vi "Turret Controller.vi"(8 "error in":errorcluster) -> ()   [LabVIEW 2019]
doc: "This VI executes continuously carrying out the current operation and responding to updates or new operations. It will often contain the timing or control code that is difficult to place directly in TeleOp. This VI generally opens all sensors and motors and isolates the rest of the robot code from knowing how the operations are carried out."
uses:
  <vilib>/Rock Robotics/WPI/Framework/Completion Status.ctl
  Turret Setpoints.ctl
  Turret Operations.ctl
  <vilib>/Rock Robotics/SystemInterfaces/DIO/FPGA_DIOChannel.ctl
  <vilib>/Rock Robotics/WPI/ThirdParty/REV Robotics/SPARK MAX/Typedef/Spark MAX Control Type.ctl
  Turret Published Globals.vi
  Framework/Robot Global Data.vi
  <vilib>/addons/control/pid/pid.llb/PID (DBL).vi
  <vilib>/addons/control/pid/NI_PID_pid.lvlib
  <vilib>/Rock Robotics/Network Tables/NT Write Boolean.vi
panel:
  out "Sensor Position 2":dbl
  out "Hood Position":T1(graph)
  out "Sensor Position":dbl
  out "Turret Position":T1(graph)
  out "Turret Position":cluster{"output":dbl, "Horizontal Offset":dbl}(graph)
  in  "DIO Channels":cluster{"Turret Encoder":T2, "Hood Encoder":T2}={"Turret Encoder"=enum."DIO 0", "Hood Encoder"=enum."DIO 1"}
  in  "Motor CAN IDs":T3={"Shooter Left"=12, "Shooter Right"=13, "Turret"=10, "Hood"=14}
  out "Setpoints":T4(graph)
  in  "Interactive Values":T5
  out "Current\nCmd":string
  in  "Buttons":cluster{"Execute Cmd":bool, "Abort Cmd":bool}
  out "Command Timing":cluster{"Start Time (ms)":u32, "Iterations":i32}
  out "Status":T7
  # "Interactive Command: You may fill in the settings for a command\nand schedule it with the Execute button. You can observe and abort\nany command while fine tuning the code for the controller."
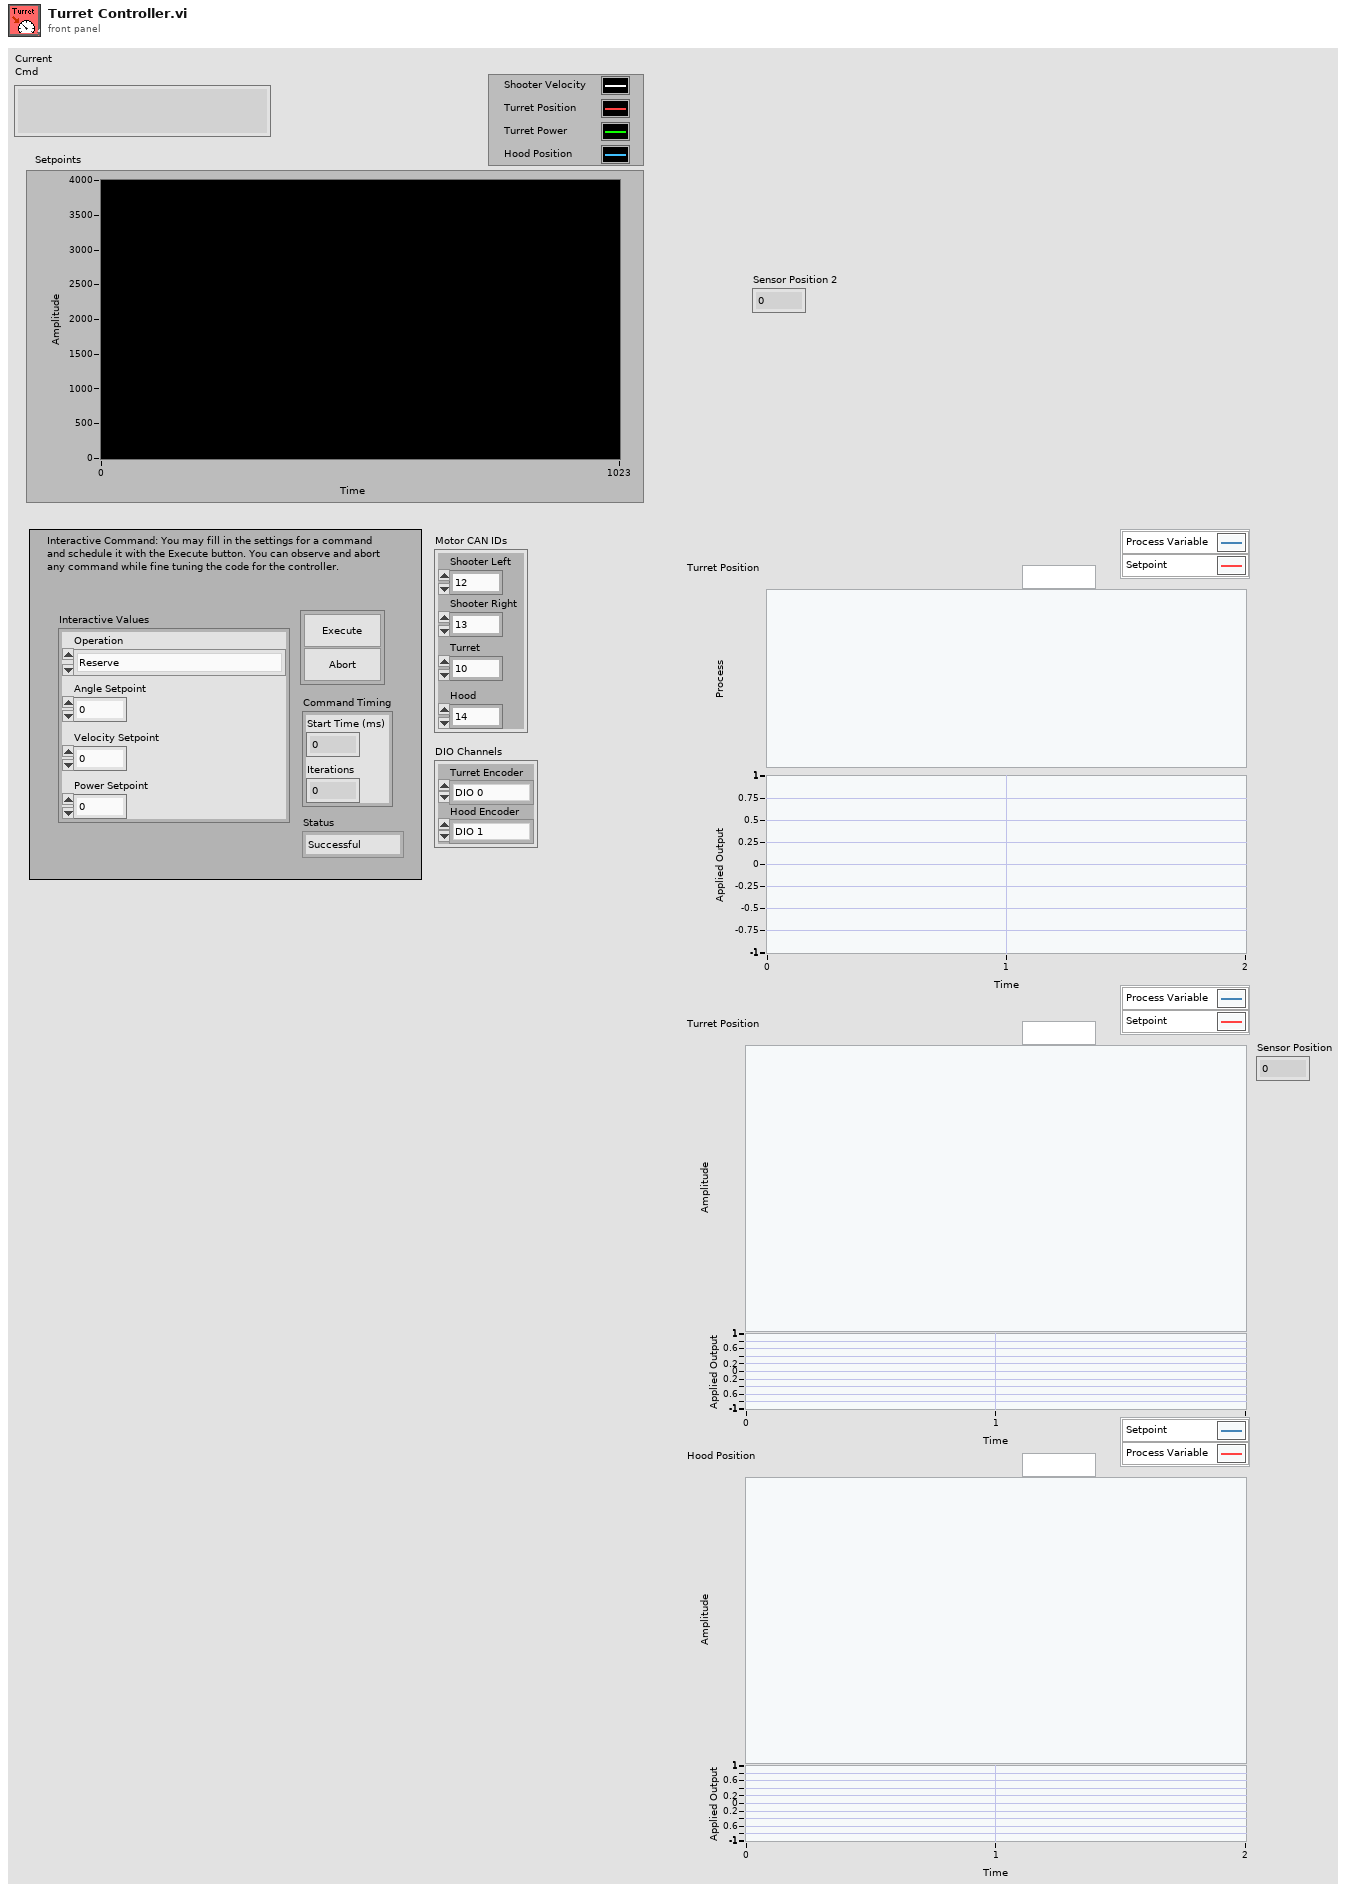
[diagram p1: front panel]
types:
  T1 = cluster{"Sensor Velocity":dbl, "Setpoint":dbl, "Applied Output":dbl}
  T2 = typedef "FPGA_DIOChannel.ctl" = enum8{"DIO 0", "DIO 1", "DIO 2", "DIO 3", "DIO 4", "DIO 5", "DIO 6", "DIO 7", "DIO 8", "DIO 9", "DIO MXP 0", "DIO MXP 1", "DIO MXP 2", "DIO MXP 3", "DIO MXP 4", "DIO MXP 5", "DIO MXP 6", "DIO MXP 7", "DIO MXP 8", "DIO MXP 9", "DIO MXP 10", "DIO MXP 11", "DIO MXP 12", "DIO MXP 13", "DIO MXP 14", "DIO MXP 15", "SPI Port CS1", "SPI Port CS2", "SPI Port CS3", "SPI Port MISO", "SPI Port MOSI", "Invalid"}
  T3 = cluster{"Shooter Left":u8, "Shooter Right":u8, "Turret":u8, "Hood":u8}
  T4 = cluster{"Velocity Setpoint":dbl, "Power Setpoint":dbl, "output":dbl, "output 2":dbl}
  T5 = typedef "Turret Setpoints.ctl" = cluster{"Operation":T6, "Angle Setpoint":dbl, "Velocity Setpoint":dbl, "Power Setpoint":dbl}
  T6 = typedef "Turret Operations.ctl" = enum16{"Reserve", "Read Current", "Immediate", "Rotate to Angle", "Align with Target", "Rotate Right Immediate", "Rotate Left Immediate", "Start Shooter", "Stop Shooter", "Lift to Angle", "Lower Immediate", "Lift Immediate"}
  T7 = typedef "Completion Status.ctl" = enum16{"Successful", "Aborted", "Incomplete"}
  T8 = typedef "WPI_MotorControlDeviceRef.ctl" = cluster{"DeviceStatus":errorcluster, "Type":T9, "PWM":cluster{"PWM Channel":T10, "DeadBand":T11}, "CAN":cluster{"Device Number":u8, "SetOutput VI Ref":variant, "GetOutput VI Ref":variant, "Enable VI Ref":variant, "Disable VI Ref":variant, "Data":variant}, "Invert":bool, "DIO PWM":cluster{"PWM \"Enable\" Channel":T10, "DIOChannel":T2, "PWM Rate":dbl}}
  T9 = typedef "WPI_MotorControlType.ctl" = enum16{"PWM", "CAN", "DIO PWM"}
  T10 = typedef "FPGA_DIOPWMChannel.ctl" = enum8{"PWM 0", "PWM 1", "PWM 2", "PWM 3", "PWM 4", "PWM 5", "PWM 6", "PWM 7", "PWM 8", "PWM 9", "PWM MXP 0", "PWM MXP 1", "PWM MXP 2", "PWM MXP 3", "PWM MXP 4", "PWM MXP 5", "PWM MXP 6", "PWM MXP 7", "PWM MXP 8", "PWM MXP 9", "Invalid"}
  T11 = typedef "WPI_PWMDeadband.ctl" = cluster{"Name":string, "maxPositivePwm":i32, "minPositivePwm":i32, "centerPwm":i32, "maxNegativePwm":i32, "minNegativePwm":i32, "angularRange":u16}
  T12 = typedef "Command Status Info.ctl" = cluster{"Name":string, "Status":T7, "notifier out":T13}
  T13 = typedef "Completion Notifier.ctl" = refnum<notifier>
  T14 = cluster{"Current Command":T5, "Command Timing":cluster{"Start Time (ms)":u32, "Iterations":i32}, "Command Arguments":cluster{"Command Info":T12, "Description":string, "Default Command":T5, "queue out":refnum<queue>, "Subsystem Name":string}}
  T15 = typedef "Spark MAX Control Type.ctl" = enum16{"Percent VBus", "Voltage", "Velocity", "Position", "Smart Motion", "Current", "Smart Velocity"}
  T16 = cluster{"Shooter Velocity":dbl, "Turret Position":dbl, "Turret Power":dbl, "Hood Position":dbl}
  T17 = cluster{"P Gain":dbl, "I Gain":dbl, "D Gain":dbl, "F Gain":dbl, "I Zone":dbl, "Min Output":dbl, "Max Output":dbl}
  T18 = cluster{"Sensor Velocity":dbl, "Shooter Velocity Setpoint":dbl, "Applied Output":dbl}
  T19 = cluster{"Valid Target":bool, "Horizontal Offset":dbl, "Vertical Offset":dbl, "Target Area":dbl, "Skew":dbl}
  T20 = cluster{"proportional gain (Kc)":dbl, "integral time (Ti, min)":dbl, "derivative time (Td, min)":dbl}
  T21 = typedef "Spark MAX Status 0 Frame.ctl" = cluster{"Applied Output":dbl, "Faults":T22, "Sticky Faults":T22, "Rsvd":u8, "Status 0 Flags":T23, "Timestamp":u32}
  T22 = typedef "Spark MAX Faults.ctl" = cluster{"Hard Limit Rev":bool, "Hard Limit Fwd":bool, "Soft Limit Fwd":bool, "Soft Limit Rev":bool, "Other Fault":bool, "DRV Fault":bool, "Has Reset?":bool, "CAN RX":bool, "CAN TX":bool, "EEPROM CRC":bool, "Stall":bool, "Sensor Fault":bool, "Motor Type Fault":bool, "IWDT Reset":bool, "Over Current":bool, "Brownout":bool}
  T23 = typedef "Spark MAX Status 0 Flags.ctl" = cluster{"Invert/Brake":bool, "Is Follower":bool}
  T24 = cluster{"Sensor Position":dbl, dbl, "Applied Output":dbl}
  T25 = cluster{"Sensor Velocity":dbl, "Velocity Setpoint":dbl, "Applied Output":dbl}
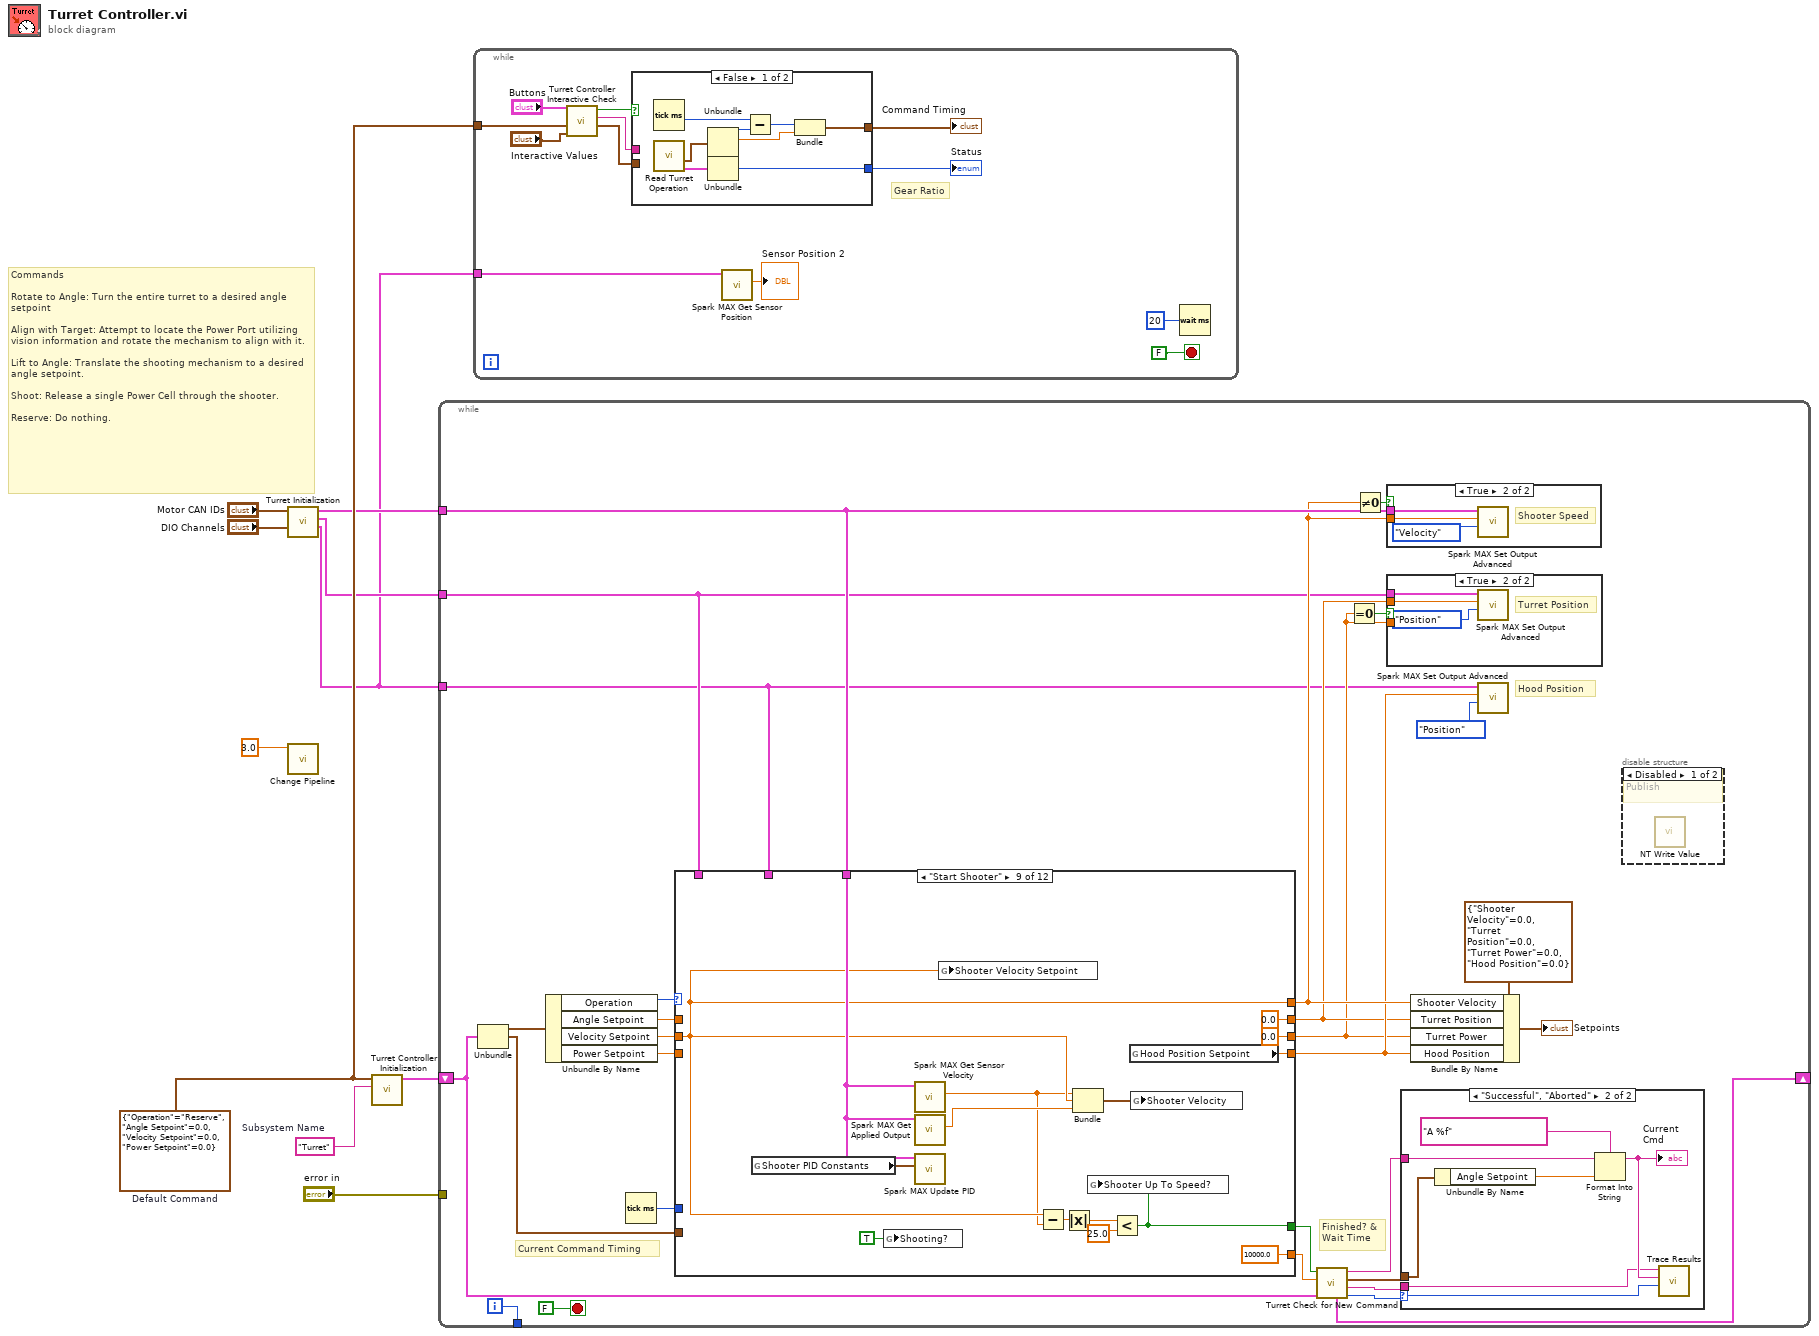
[diagram p0: block diagram]
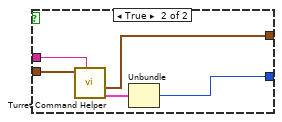
[diagram p2: hidden frame]
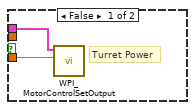
[diagram p3: hidden frame]
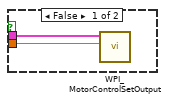
[diagram p4: hidden frame]
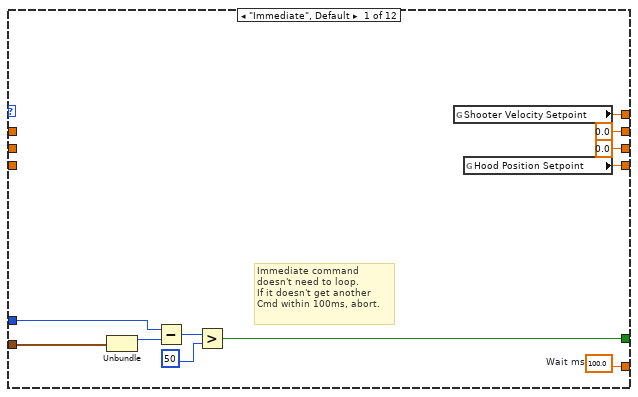
[diagram p7: hidden frame]
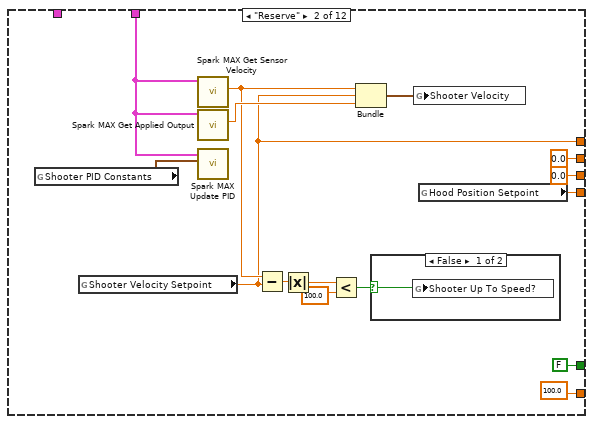
[diagram p8: hidden frame]
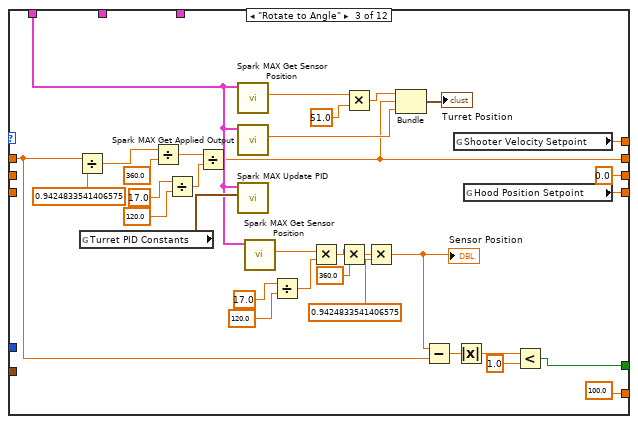
[diagram p10: hidden frame]
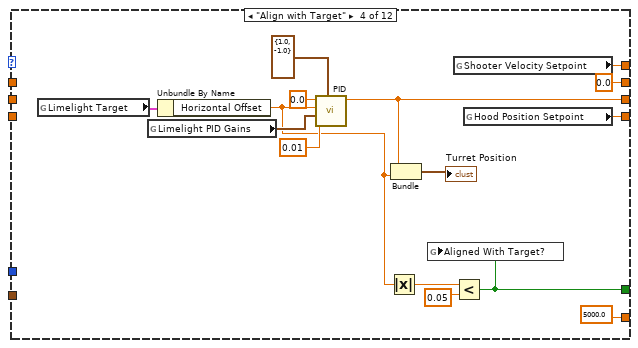
[diagram p11: hidden frame]
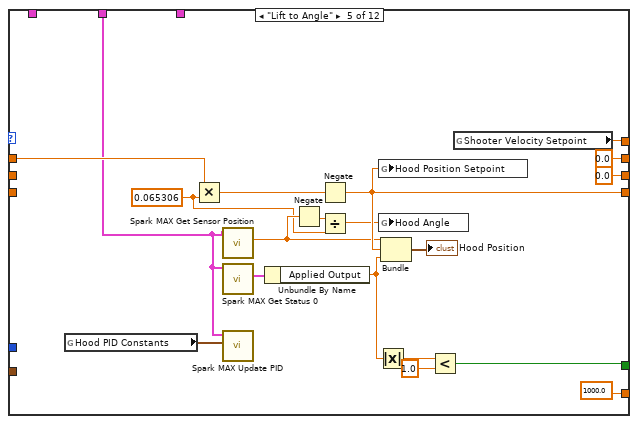
[diagram p12: hidden frame]
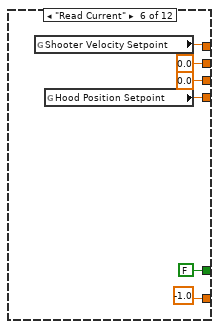
[diagram p13: hidden frame]
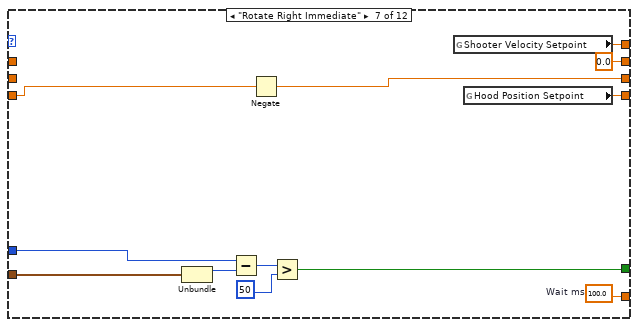
[diagram p14: hidden frame]
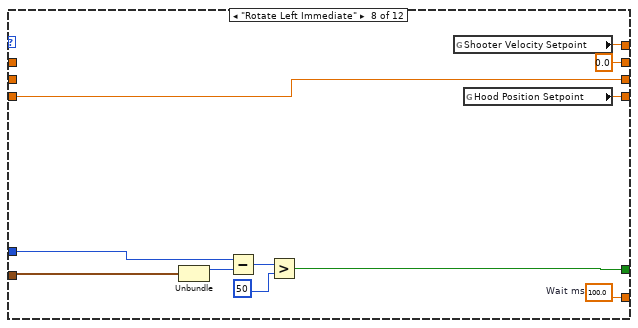
[diagram p15: hidden frame]
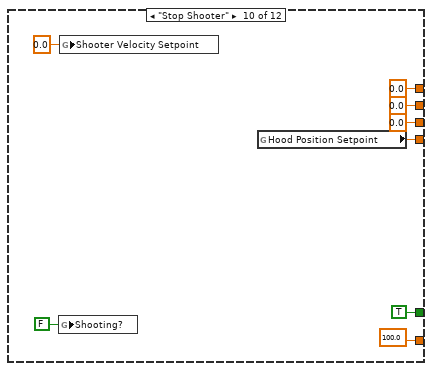
[diagram p16: hidden frame]
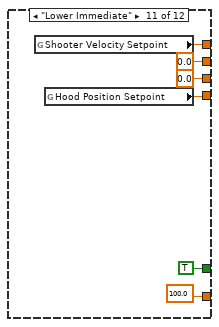
[diagram p17: hidden frame]
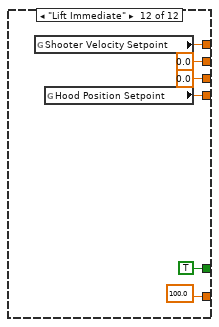
[diagram p18: hidden frame]
diagram:
  w7 = T5 {"Operation"=enum."Reserve", "Angle Setpoint"=0.0, "Velocity Setpoint"=0.0, "Power Setpoint"=0.0}  # Default Command
  w8 = "Turret"  # Subsystem Name
  # "Commands\n\nRotate to Angle: Turn the entire turret to a desired angle setpoint\n\nAlign with Target: Attempt to locate the Power Port utilizing vision information and rotate the mechanism to align with it.\n\nLift to Angle: Translate the shooting mechanism to a desired angle setpoint.\n\nShoot: Release a single Power Cell through the shooter.\n\nReserve: Do nothing."
  n1 = call "Turret Initialization.vi"("DIO Channels"="DIO Channels", "Motor CAN IDs"="Motor CAN IDs") -> ("Hood"=w1:T8, "Turret"=w3:T8, "Shooter"=w2:T8)  [unwired: 7 in]
  n2 = call "Change Pipeline.vi"("Index"=3.0) -> ()  [unwired: 11 in]
  n3 = call "Turret Controller Initialization.vi"("Subsystem Name"=w8, "Default Command"=w7) -> ("Current Command"=w9:T14)  [unwired: 9 in]
  n4 = while {
    shift-right: [w32] -> _
    shift-left: w9 -> [w25]
    tunnel: [w38] -> _
    tunnel: "error in" -> [_]
    tunnel: w2 -> [w22]
    tunnel: w3 -> [w15]
    tunnel: w1 -> [w11]
    i -> [w38]
    stop <- FALSE stop-if-true
    # "Hood Position"
    # "Current Command Timing"
    # "Finished? &\nWait Time"
    n5 = Unbundle(w25) -> ("Current Command"=w37:T5, "Command Timing"=w33:cluster{"Start Time (ms)":u32, "Iterations":i32})  [unwired: 1 out]
    n6 = Unbundle By Name(w37) -> ("Operation"=w36:T6, "Angle Setpoint"=w35:dbl, "Velocity Setpoint"=w24:dbl, "Power Setpoint"=w23:dbl)
    n7 = Tick Count (ms)() -> (millisecond timer value=w34:u32)
    n8 = case shown="\"Start Shooter\"" w36 {
      tunnel: [w67 100.0 ("Wait ms") 100.0 ("Wait ms") 5000.0 ("Infinite") 1000.0 ("Infinite") -1.0 ("Infinite") w163 w175 10000.0 ("Wait ms") 100.0 ("Wait ms") 100.0 ("Wait ms") 100.0 ("Wait ms")] -> w30
      tunnel: [w61 FALSE ("ignore previous (F)") w98 w121 w133 FALSE ("ignore previous (F)") w162 w176 w191 TRUE ("ignore previous (F)") TRUE ("ignore previous (F)") TRUE ("ignore previous (F)")] -> w31
      tunnel: w33 -> [w63 _ _ _ _ _ w164 w173 _ _ _ _]
      tunnel: w35 -> [_ _ w85 _ w149 _ _ _ _ _ _ _]
      tunnel: w34 -> [w62 _ _ _ _ _ w165 w174 _ _ _ _]
      tunnel: w24 -> [_ _ _ _ _ _ _ _ w190 _ _ _]
      tunnel: [w60 w68 w114 w130 w144 w154 w161 w172 w190 0.0 ("Shooter Velocity Setpoint") w206 w212] -> w20
      tunnel: [0.0 ("Power Setpoint") 0.0 ("Power Setpoint") w101 0.0 ("Power Setpoint") 0.0 ("Power Setpoint") 0.0 ("Power Setpoint") 0.0 ("Power Setpoint") 0.0 ("Power Setpoint") 0.0 ("Power Setpoint") 0.0 ("Power Setpoint") 0.0 ("Power Setpoint") 0.0 ("Power Setpoint")] -> w16
      tunnel: w23 -> [_ _ _ _ _ _ w158 w170 _ _ _ _]
      tunnel: [0.0 ("output") 0.0 ("output") 0.0 ("output") w120 0.0 ("output") 0.0 ("output") w159 w170 0.0 ("output") 0.0 ("output") 0.0 ("output") 0.0 ("output")] -> w13
      tunnel: w11 -> [_ _ _ _ w138 _ _ _ _ _ _ _]
      tunnel: [w59 w80 w113 w119 w142 w152 w160 w171 w189 w197 w205 w211] -> w19
      tunnel: w22 -> [_ w75 _ _ _ _ _ _ w192 _ _ _]
      tunnel: w15 -> [_ _ w109 _ _ _ _ _ _ _ _ _]
      frame "Immediate", Default {
        w67 = 100.0  # Wait ms
        # "Immediate command\ndoesn't need to loop.\nIf it doesn't get another\nCmd within 100ms, abort."
        n9 = Unbundle(w63) -> ("Start Time (ms)"=w66:u32)  [unwired: 1 out]
        n10 = Subtract(x=w62, y=w66) -> (x-y=w65:u32)
        n11 = Greater?(x=w65, y=u8 50 ("Left Motor")) -> (0:w61:bool)
        n12 = global read "Turret Published Globals.vi" "Shooter Velocity Setpoint"() -> (w60:dbl)
        n13 = global read "Turret Published Globals.vi" "Hood Position Setpoint"() -> (w59:dbl)
      }
      frame "Reserve" {
        n14 = global read "Turret Published Globals.vi" "Shooter PID Constants"() -> (w76:T17)
        n15 = global read "Turret Published Globals.vi" "Shooter Velocity Setpoint"() -> (w68:dbl)
        n16 = call <vilib>:"Spark MAX Get Sensor Velocity.vi"("MotorControlDevRef in"=w75) -> ("Sensor Velocity"=w71:dbl)  [unwired: 7 in, 3 out]
        n17 = call <vilib>:"Spark MAX Get Applied Output.vi"("MotorControlDevRef in"=w75) -> ("Applied Output"=w77:dbl)  [unwired: 7 in, 3 out]
        n18 = call "Spark MAX Update PID.vi"("MotorControlDeviceRef"=w75, "PID Constants"=w76) -> ()  [unwired: 8 in]
        n19 = Subtract(x=w71, y=w68) -> (x-y=w74:dbl)
        n20 = Absolute Value(x=w74) -> (abs(x)=w73:dbl)
        n21 = Less?(x=w73, y=100.0) -> (x < y?=w70:bool)
        n22 = Bundle("Sensor Velocity"=w71, "Shooter Velocity Setpoint"=w68, "Applied Output"=w77) -> (w78:T18)  [unwired: 1 in]
        n23 = case shown="False" w70 {
          selector: w70 -> [w83 _]
          frame False {
            n24 = global write "Turret Published Globals.vi" "Shooter Up To Speed?"(w83) -> ()
          }
          frame True {
          }
        }
        n25 = global write "Turret Published Globals.vi" "Shooter Velocity"(w78) -> ()
        n26 = global read "Turret Published Globals.vi" "Hood Position Setpoint"() -> (w80:dbl)
      }
      frame "Rotate to Angle" {
        n27 = Divide(x=w85, y=0.9424833541406575) -> (x/y=w100:dbl)
        n28 = global read "Turret Published Globals.vi" "Turret PID Constants"() -> (w115:T17)
        n29 = Divide(x=w100, y=360.0) -> (x/y=w102:dbl)
        n30 = Divide(x=17.0, y=120.0) -> (x/y=w107:dbl)
        n31 = Divide(x=w102, y=w107) -> (x/y=w101:dbl)
        n32 = call <vilib>:"Spark MAX Get Sensor Position.vi"("MotorControlDevRef in"=w109) -> ("Sensor Position"=w112:dbl)  [unwired: 7 in, 3 out]
        n33 = call <vilib>:"Spark MAX Get Applied Output.vi"("MotorControlDevRef in"=w109) -> ("Applied Output"=w108:dbl)  [unwired: 7 in, 3 out]
        n34 = call "Spark MAX Update PID.vi"("MotorControlDeviceRef"=w109, "PID Constants"=w115) -> ()  [unwired: 8 in]
        n35 = call <vilib>:"Spark MAX Get Sensor Position.vi"("MotorControlDevRef in"=w109) -> ("Sensor Position"=w92:dbl)  [unwired: 7 in, 3 out]
        n36 = Divide(x=17.0, y=120.0) -> (x/y=w91:dbl)
        n37 = Multiply(x=w92, y=w91) -> (x*y=w90:dbl)
        n38 = Multiply(x=w90, y=360.0) -> (x*y=w88:dbl)
        n39 = Multiply(x=w112, y=51.0) -> (x*y=w110:dbl)
        n40 = Multiply(x=w88, y=0.9424833541406575) -> (x*y=w86:dbl)
        "Sensor Position" <- w86
        n41 = Bundle(w110, w101, "Applied Output"=w108) -> (→"Turret Position":cluster{dbl, dbl, "Applied Output":dbl})  [unwired: 1 in]
        n42 = Subtract(x=w86, y=w85) -> (x-y=w97:dbl)
        n43 = global read "Turret Published Globals.vi" "Shooter Velocity Setpoint"() -> (w114:dbl)
        n44 = Absolute Value(x=w97) -> (abs(x)=w96:dbl)
        n45 = global read "Turret Published Globals.vi" "Hood Position Setpoint"() -> (w113:dbl)
        n46 = Less?(x=w96, y=1.0) -> (x < y?=w98:bool)
      }
      frame "Align with Target" {
        n47 = global read "Robot Global Data.vi" "Limelight Target"() -> (w129:T19)
        n48 = global read "Turret Published Globals.vi" "Limelight PID Gains"() -> (w126:T20)
        n49 = Unbundle By Name(w129) -> ("Horizontal Offset"=w118:dbl)
        n50 = call-poly <vilib>:"PID.vi"("output range"=cluster{"output high":dbl, "output low":dbl} {"output high"=1.0, "output low"=-1.0}, "dt (s)"=0.01, "PID gains"=w126, "process variable"=w118, "setpoint"=0.0) -> ("output"=w120:dbl)  [unwired: 5 in, 1 out]
        n51 = Absolute Value(x=w118) -> (abs(x)=w123:dbl)
        n52 = Bundle("output"=w120, "Horizontal Offset"=w118) -> (→"Turret Position":cluster{"output":dbl, "Horizontal Offset":dbl})  [unwired: 1 in]
        n53 = global read "Turret Published Globals.vi" "Shooter Velocity Setpoint"() -> (w130:dbl)
        n54 = Less?(x=w123, y=0.05) -> (x < y?=w121:bool)
        n55 = global write "Turret Published Globals.vi" "Aligned With Target?"(w121) -> ()
        n56 = global read "Turret Published Globals.vi" "Hood Position Setpoint"() -> (w119:dbl)
      }
      frame "Lift to Angle" {
        w135 = 0.065306 ("y")
        n57 = global read "Turret Published Globals.vi" "Hood PID Constants"() -> (w145:T17)
        n58 = Multiply(x=w149, y=w135) -> (x*y=w148:dbl)
        n59 = call <vilib>:"Spark MAX Get Sensor Position.vi"("MotorControlDevRef in"=w138) -> ("Sensor Position"=w137:dbl)  [unwired: 7 in, 3 out]
        n60 = call <vilib>:"Spark MAX Get Status 0.vi"("MotorControlDevRef"=w138) -> ("Status 0"=w147:T21)  [unwired: 7 in, 3 out]
        n61 = call "Spark MAX Update PID.vi"("MotorControlDeviceRef"=w138, "PID Constants"=w145) -> ()  [unwired: 8 in]
        n62 = Unbundle By Name(w147) -> ("Applied Output"=w139:dbl)
        n63 = Negate(x=w137) -> (-x=w136:dbl)
        n64 = Negate(x=w148) -> (-x=w142:dbl)
        n65 = Divide(x=w136, y=w135) -> (x/y=w134:dbl)
        n66 = Absolute Value(x=w139) -> (abs(x)=w140:dbl)
        n67 = global write "Turret Published Globals.vi" "Hood Position Setpoint"(w142) -> ()
        n68 = global write "Turret Published Globals.vi" "Hood Angle"(w134) -> ()
        n69 = Bundle("Sensor Position"=w137, w142, "Applied Output"=w139) -> (→"Hood Position":T24)  [unwired: 1 in]
        n70 = Less?(x=w140, y=1.0) -> (x < y?=w133:bool)
        n71 = global read "Turret Published Globals.vi" "Shooter Velocity Setpoint"() -> (w144:dbl)
      }
      frame "Read Current" {
        n72 = global read "Turret Published Globals.vi" "Shooter Velocity Setpoint"() -> (w154:dbl)
        n73 = global read "Turret Published Globals.vi" "Hood Position Setpoint"() -> (w152:dbl)
      }
      frame "Rotate Right Immediate" {
        w163 = 100.0  # Wait ms
        n74 = Unbundle(w164) -> ("Start Time (ms)"=w168:u32)  [unwired: 1 out]
        n75 = Subtract(x=w165, y=w168) -> (x-y=w167:u32)
        n76 = Negate(x=w158) -> (-x=w159:dbl)
        n77 = Greater?(x=w167, y=u8 50 ("Left Motor")) -> (0:w162:bool)
        n78 = global read "Turret Published Globals.vi" "Shooter Velocity Setpoint"() -> (w161:dbl)
        n79 = global read "Turret Published Globals.vi" "Hood Position Setpoint"() -> (w160:dbl)
      }
      frame "Rotate Left Immediate" {
        w175 = 100.0  # Wait ms
        n80 = Unbundle(w173) -> ("Start Time (ms)"=w179:u32)  [unwired: 1 out]
        n81 = Subtract(x=w174, y=w179) -> (x-y=w178:u32)
        n82 = Greater?(x=w178, y=u8 50 ("Left Motor")) -> (0:w176:bool)
        n83 = global read "Turret Published Globals.vi" "Shooter Velocity Setpoint"() -> (w172:dbl)
        n84 = global read "Turret Published Globals.vi" "Hood Position Setpoint"() -> (w171:dbl)
      }
      frame "Start Shooter" {
        n85 = global read "Turret Published Globals.vi" "Shooter PID Constants"() -> (w193:T17)
        n86 = global write "Turret Published Globals.vi" "Shooting?"(TRUE ("Shooting?")) -> ()
        n87 = call <vilib>:"Spark MAX Get Sensor Velocity.vi"("MotorControlDevRef in"=w192) -> ("Sensor Velocity"=w185:dbl)  [unwired: 7 in, 3 out]
        n88 = call <vilib>:"Spark MAX Get Applied Output.vi"("MotorControlDevRef in"=w192) -> ("Applied Output"=w186:dbl)  [unwired: 7 in, 3 out]
        n89 = call "Spark MAX Update PID.vi"("MotorControlDeviceRef"=w192, "PID Constants"=w193) -> ()  [unwired: 8 in]
        n90 = global write "Turret Published Globals.vi" "Shooter Velocity Setpoint"(w190) -> ()
        n91 = Subtract(x=w190, y=w185) -> (x-y=w184:dbl)
        n92 = Absolute Value(x=w184) -> (abs(x)=w183:dbl)
        n93 = Bundle("Sensor Velocity"=w185, "Velocity Setpoint"=w190, "Applied Output"=w186) -> (w181:T25)  [unwired: 1 in]
        n94 = Less?(x=w183, y=25.0) -> (x < y?=w191:bool)
        n95 = global write "Turret Published Globals.vi" "Shooter Up To Speed?"(w191) -> ()
        n96 = global read "Turret Published Globals.vi" "Hood Position Setpoint"() -> (w189:dbl)
        n97 = global write "Turret Published Globals.vi" "Shooter Velocity"(w181) -> ()
      }
      frame "Stop Shooter" {
        n98 = global write "Turret Published Globals.vi" "Shooting?"(FALSE ("Shooting?")) -> ()
        n99 = global write "Turret Published Globals.vi" "Shooter Velocity Setpoint"(0.0 ("Shooter Velocity Setpoint")) -> ()
        n100 = global read "Turret Published Globals.vi" "Hood Position Setpoint"() -> (w197:dbl)
      }
      frame "Lower Immediate" {
        n101 = global read "Turret Published Globals.vi" "Shooter Velocity Setpoint"() -> (w206:dbl)
        n102 = global read "Turret Published Globals.vi" "Hood Position Setpoint"() -> (w205:dbl)
      }
      frame "Lift Immediate" {
        n103 = global read "Turret Published Globals.vi" "Shooter Velocity Setpoint"() -> (w212:dbl)
        n104 = global read "Turret Published Globals.vi" "Hood Position Setpoint"() -> (w211:dbl)
      }
    }
    n105 = call "Turret Check for New Command.vi"("Current Command"=w25, "Wait time (ms)"=w30, "Finished?"=w31) -> ("Completion"=w26:T7, "Subsystem Name"=w27:string, "Current Command"=w28:T5, "Initial Trace String"=w29:string, "NextCommand"=w32:T14)  [unwired: 4 in]
    n106 = Equal To 0?(x=w13) -> (x = 0?=w14:bool)
    n107 = Not Equal To 0?(x=w20) -> (x != 0?=w21:bool)
    n108 = case shown="True" w21 {
      tunnel: w22 -> [w46 w48]
      tunnel: w20 -> [w45 w47]
      frame False {
        n109 = call <vilib>:"WPI_MotorControlSetOutput.vi"("Output"=w45, "MotorControlDevRef"=w46) -> ()  [unwired: 7 in, 3 out]
      }
      frame True {
        # "Shooter Speed"
        n110 = call <vilib>:"Spark MAX Set Output Advanced.vi"("Control Mode"=Spark_MAX_Control_Type."Velocity", "Setpoint"=w47, "MotorControlDevRef"=w48) -> ()  [unwired: 7 in, 2 out]
      }
    }
    n111 = case shown="True" w14 {
      tunnel: w16 -> [_ w43]
      tunnel: w15 -> [w40 w42]
      tunnel: w13 -> [w41 _]
      frame False {
        # "Turret Power"
        n112 = call <vilib>:"WPI_MotorControlSetOutput.vi"("Output"=w41, "MotorControlDevRef"=w40) -> ()  [unwired: 7 in, 3 out]
      }
      frame True {
        # "Turret Position"
        n113 = call <vilib>:"Spark MAX Set Output Advanced.vi"("Control Mode"=Spark_MAX_Control_Type."Position", "Setpoint"=w43, "MotorControlDevRef"=w42) -> ()  [unwired: 7 in, 2 out]
      }
    }
    n114 = case shown="\"Successful\", \"Aborted\"" w26 {
      selector: w26 -> [_ w56]
      tunnel: w29 -> [_ w52]
      tunnel: w28 -> [_ w53]
      tunnel: w27 -> [_ w50]
      frame "Incomplete", Default {
        # "Continuing current command"
      }
      frame "Successful", "Aborted" {
        # "Report and setup for next command"
        n115 = Unbundle By Name(w53) -> ("Angle Setpoint"=w55:dbl)
        n116 = Format Into String(format string="A %f", initial string=w52, w55) -> (resulting string=w51:string)  [unwired: 1 in, 1 out]
        "Current\nCmd" <- w51
        n117 = call <vilib>:"Trace Results.vi"("Status of previous command"=w56, "Description"=w51, "Subsystem"=w50) -> ()  [unwired: 9 in]
      }
    }
    n118 = Bundle By Name(cluster=T16 {"Shooter Velocity"=0.0, "Turret Position"=0.0, "Turret Power"=0.0, "Hood Position"=0.0} ("Setpoints"), "Shooter Velocity"=w20, "Turret Position"=w16, "Turret Power"=w13, "Hood Position"=w19) -> (→"Setpoints":T16)
    n119 = call <vilib>:"Spark MAX Set Output Advanced.vi"("Control Mode"=Spark_MAX_Control_Type."Position", "Setpoint"=w19, "MotorControlDevRef"=w11) -> ()  [unwired: 7 in, 2 out]
    n120 = disable-structure shown="Disabled" {
      frame Disabled {
        # "Publish"
        n121 = call-poly <vilib>:"NT Write Value.vi"() -> ()  [unwired: 11 in, 1 out]
      }
      frame Enabled {
      }
    }
  }
  n122 = while {
    tunnel: w7 -> [w223]
    tunnel: w1 -> [w215]
    stop <- FALSE stop-if-true
    # "Gear Ratio"
    n123 = call "Turret Controller Interactive Check.vi"("Interactive Command in"="Interactive Values", "Default Command"=w223, "Buttons"="Buttons") -> ("Interactive Command out"=w220:T5, "Trace String"=w221:string, "Schedule"=w222:bool)  [unwired: 6 in]
    n124 = case shown="False" w222 {
      tunnel: [w234 w239] -> w219
      tunnel: w220 -> [_ w237]
      tunnel: [w230 w235] -> w218
      tunnel: w221 -> [_ w238]
      frame False {
        n125 = Tick Count (ms)() -> (millisecond timer value=w229:u32)
        n126 = call "Read Turret Operation.vi"() -> ("Command Info"=w227:T12, "SubSystem Data"=w228:T5)  [unwired: 9 in, 1 out]
        n127 = Unbundle(w228) -> ("Operation"=w233:T6, "Angle Setpoint"=w231:dbl)  [unwired: 2 out]
        n128 = Unbundle(w227) -> ("Status"=w234:T7)  [unwired: 2 out]
        n129 = Subtract(x=w229, y=w233) -> (x-y=w232:u32)
        n130 = Bundle(w232, "Angle Setpoint"=w231) -> (w230:cluster{u32, "Angle Setpoint":dbl})  [unwired: 1 in]
      }
      frame True {
        n131 = call "Turret Command Helper.vi"("Description"=w238, "SubSystem Data"=w237) -> ("Command Info Out"=w236:T12, "Command Timing"=w235:cluster{"Start Time (ms)":u32, "Iterations":i32})  [unwired: 7 in, 1 out]
        n132 = Unbundle(w236) -> ("Status"=w239:T7)  [unwired: 2 out]
      }
    }
    "Status" <- w219
    "Command Timing" <- w218
    n133 = call <vilib>:"Spark MAX Get Sensor Position.vi"("MotorControlDevRef in"=w215) -> ("Sensor Position"=→"Sensor Position 2":dbl)  [unwired: 7 in, 3 out]
    n134 = Wait (ms)(milliseconds to wait=u32 20) -> ()  [unwired: 1 out]
  }
